vi "Tag initialize.vi"() -> (9 "Alarm tag":refnum<class "NI Skyline Tag.lvclass">, 11 "Table tag":refnum<class "NI Skyline Tag.lvclass">, 13 "Button tag":refnum<class "NI Skyline Tag.lvclass">, 14 "RMS tag":refnum<class "NI Skyline Tag.lvclass">, 15 "RPM tag":refnum<class "NI Skyline Tag.lvclass">, 16 "Voltage tag":refnum<class "NI Skyline Tag.lvclass">, 17 "Current Tag":refnum<class "NI Skyline Tag.lvclass">, 18 "Temper tag":refnum<class "NI Skyline Tag.lvclass">, 19 "error out":errorcluster)   [LabVIEW 2017]
uses:
  <vilib>/Skyline/Tag/Wrapper/Wrapper_class/NI Skyline Tag.lvclass
  <vilib>/Skyline/Tag/Shared/typedefs/DataType.ctl
  <vilib>/Skyline/Tag/Wrapper/Wrapper AMQP_class/Open Tag AMQP.vi
  <vilib>/Skyline/Tag/Wrapper/Wrapper AMQP_class/NI Skyline Tag AMQP.lvclass
  <vilib>/Skyline/Tag/Shared/NI Skyline Tag.lvlib
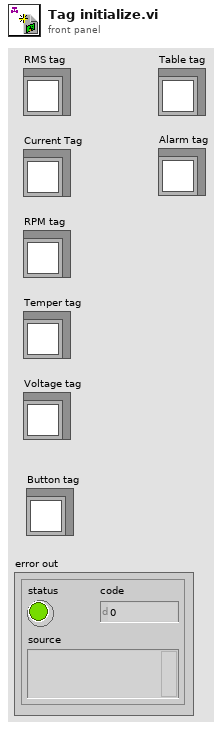
[diagram p1: front panel]
types:
  T1 = typedef "NI Skyline Tag.lvlib/DataType.ctl" = enum32{"Double", "I32", "String", "Boolean", "U64", "Timestamp"}
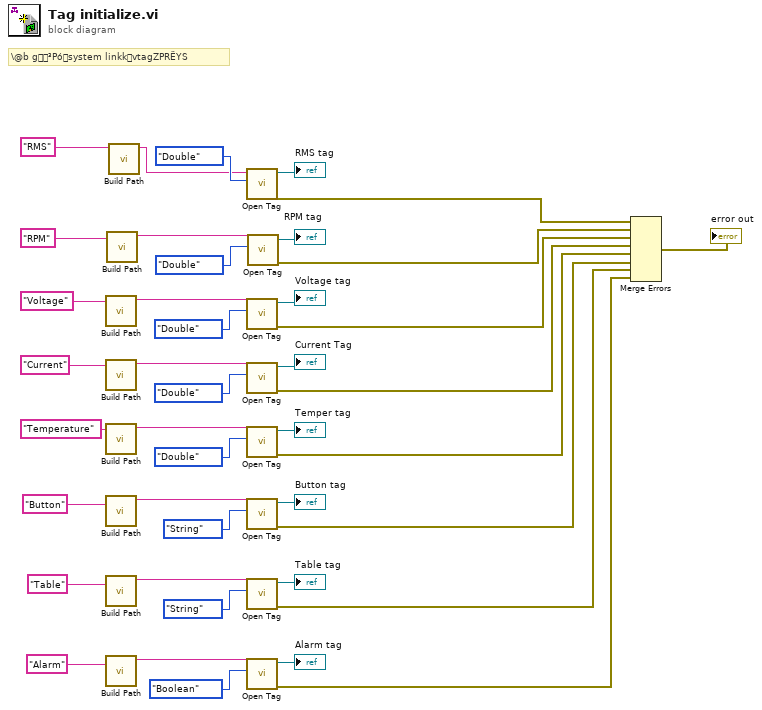
[diagram p0: block diagram]
diagram:
  # "\\@b\tg³Pósystem linkkvtagZPRËYS"
  n1 = call <vilib>:"Build Path.vi"("tag name"="Voltage" ("tag path")) -> ("path"=w24:string)  [unwired: 10 in]
  n2 = call <vilib>:"Build Path.vi"("tag name"="Current" ("tag path")) -> ("path"=w29:string)  [unwired: 10 in]
  n3 = call <vilib>:"Build Path.vi"("tag name"="Temperature" ("tag path")) -> ("path"=w30:string)  [unwired: 10 in]
  n4 = call <vilib>:"Build Path.vi"("tag name"="Button" ("tag path")) -> ("path"=w15:string)  [unwired: 10 in]
  n5 = call <vilib>:"Build Path.vi"("tag name"="Table" ("tag path")) -> ("path"=w7:string)  [unwired: 10 in]
  n6 = call <vilib>:"Build Path.vi"("tag name"="Alarm" ("tag path")) -> ("path"=w5:string)  [unwired: 10 in]
  n7 = call <vilib>:"Build Path.vi"("tag name"="RPM" ("tag path")) -> ("path"=w22:string)  [unwired: 10 in]
  n8 = call <vilib>:"Build Path.vi"("tag name"="RMS" ("tag path")) -> ("path"=w20:string)  [unwired: 10 in]
  n9 = call-poly <vilib>:"Open Tag.vi"("data type"=DataType."Double" ("Data Type"), "path"=w20) -> ("error out"=w16:errorcluster, "tag out"=→"RMS tag":refnum<class "NI Skyline Tag.lvclass">)  [unwired: 8 in]
  n10 = call-poly <vilib>:"Open Tag.vi"("data type"=DataType."Double" ("Data Type"), "path"=w24) -> ("error out"=w33:errorcluster, "tag out"=→"Voltage tag":refnum<class "NI Skyline Tag.lvclass">)  [unwired: 8 in]
  n11 = call-poly <vilib>:"Open Tag.vi"("data type"=DataType."Double" ("Data Type"), "path"=w29) -> ("error out"=w34:errorcluster, "tag out"=→"Current Tag":refnum<class "NI Skyline Tag.lvclass">)  [unwired: 8 in]
  n12 = call-poly <vilib>:"Open Tag.vi"("data type"=DataType."Double" ("Data Type"), "path"=w30) -> ("error out"=w35:errorcluster, "tag out"=→"Temper tag":refnum<class "NI Skyline Tag.lvclass">)  [unwired: 8 in]
  n13 = call-poly <vilib>:"Open Tag.vi"("data type"=DataType."String" ("Data Type"), "path"=w15) -> ("error out"=w11:errorcluster, "tag out"=→"Button tag":refnum<class "NI Skyline Tag.lvclass">)  [unwired: 8 in]
  n14 = call-poly <vilib>:"Open Tag.vi"("data type"=DataType."String" ("Data Type"), "path"=w7) -> ("error out"=w6:errorcluster, "tag out"=→"Table tag":refnum<class "NI Skyline Tag.lvclass">)  [unwired: 8 in]
  n15 = call-poly <vilib>:"Open Tag.vi"("data type"=DataType."Boolean" ("Data Type"), "path"=w5) -> ("error out"=w1:errorcluster, "tag out"=→"Alarm tag":refnum<class "NI Skyline Tag.lvclass">)  [unwired: 8 in]
  n16 = call-poly <vilib>:"Open Tag.vi"("data type"=DataType."Double" ("Data Type"), "path"=w22) -> ("error out"=w17:errorcluster, "tag out"=→"RPM tag":refnum<class "NI Skyline Tag.lvclass">)  [unwired: 8 in]
  n17 = Merge Errors(w16, w17, w33, w34, w35, w11, w6, w1) -> (→"error out":errorcluster)
